vi "BLM Move.vi"(1 "Mode IS:":bool, 2 "Steps/rot":dbl=8000.0, 3 "error in (no error)":errorcluster, 4 "Position / Distance":dbl=1.0 min=-193273528.32 max=193273528.0 step=0.09 format="%.2f", 5 "Motor Address":string="0", 6 "Port Address":refnum<visa-resource-name>) -> (0 "error out":errorcluster)   [LabVIEW 2019]
panel:
  out "Command string":string
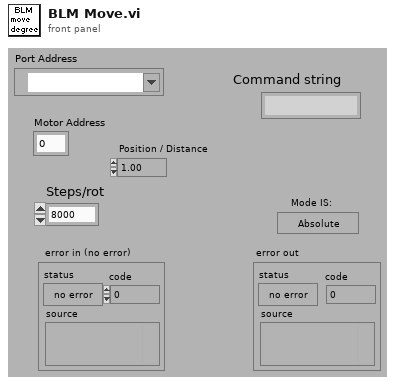
[diagram p1: front panel]
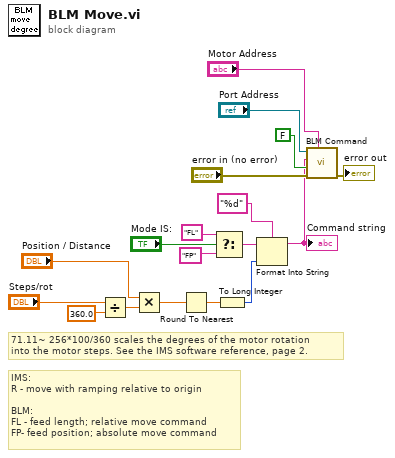
[diagram p0: block diagram]
diagram:
  # "IMS:\nR - move with ramping relative to origin\n\nBLM:\nFL - feed length; relative move command\nFP- feed position; absolute move command"
  # "71.11~ 256*100/360 scales the degrees of the motor rotation\ninto the motor steps. See the IMS software reference, page 2."
  n1 = Divide(x="Steps/rot", y=360.0) -> (x/y=w6:dbl)
  n2 = Multiply(x="Position / Distance", y=w6) -> (x*y=w16:dbl)
  n3 = Round To Nearest(number=w16) -> (nearest integer value=w15:dbl)
  n4 = Select(t="FL", s="Mode IS:", f="FP") -> (s? t:f=w10:string)
  n5 = To Long Integer(number=w15) -> (32bit integer=w7:i32)
  n6 = Format Into String(format string="%d", initial string=w10, w7) -> (resulting string=w9:string)  [unwired: 1 in, 1 out]
  "Command string" <- w9
  n7 = call "BLM Command.vi"("Motor Address"="Motor Address", "error in (no error)"="error in (no error)", "Read Echo?"=FALSE, "Command"=w9, "Port Address"="Port Address") -> ("error out"=→"error out":errorcluster)  [unwired: 1 in, 4 out]
